vi "Calc.vi"(1 "y":sgl, 2 "x":sgl, 3 "X_r":dbl, 4 "X_l":dbl) -> ()   [LabVIEW 2012]
panel:
  out "Found?":bool
  out "MC":dbl
  out "gamma (deg)":dbl
  out "gamma (rad)":dbl
  out "MF":dbl
  in  "Set Distance [m]":dbl
  out "Beta (angle to target) [deg]":dbl
  out "cos_2alpha":dbl
  out "F_1B_1":i32
  out "s":dbl
  out "A_1F":dbl
  out "A_1B_1":dbl
  out "F_1A_1":i32
  out "Beta (rad)":dbl
  out "CF (distance to target) [m]":dbl
  # "Input"
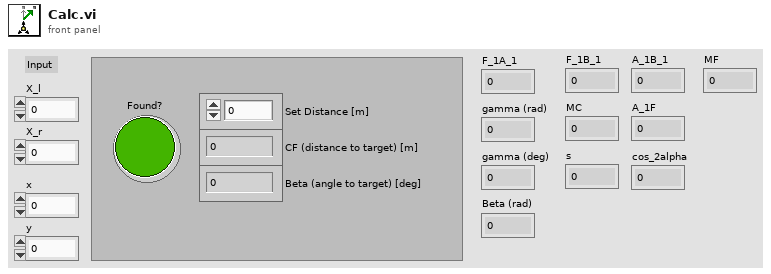
[diagram p1: front panel]
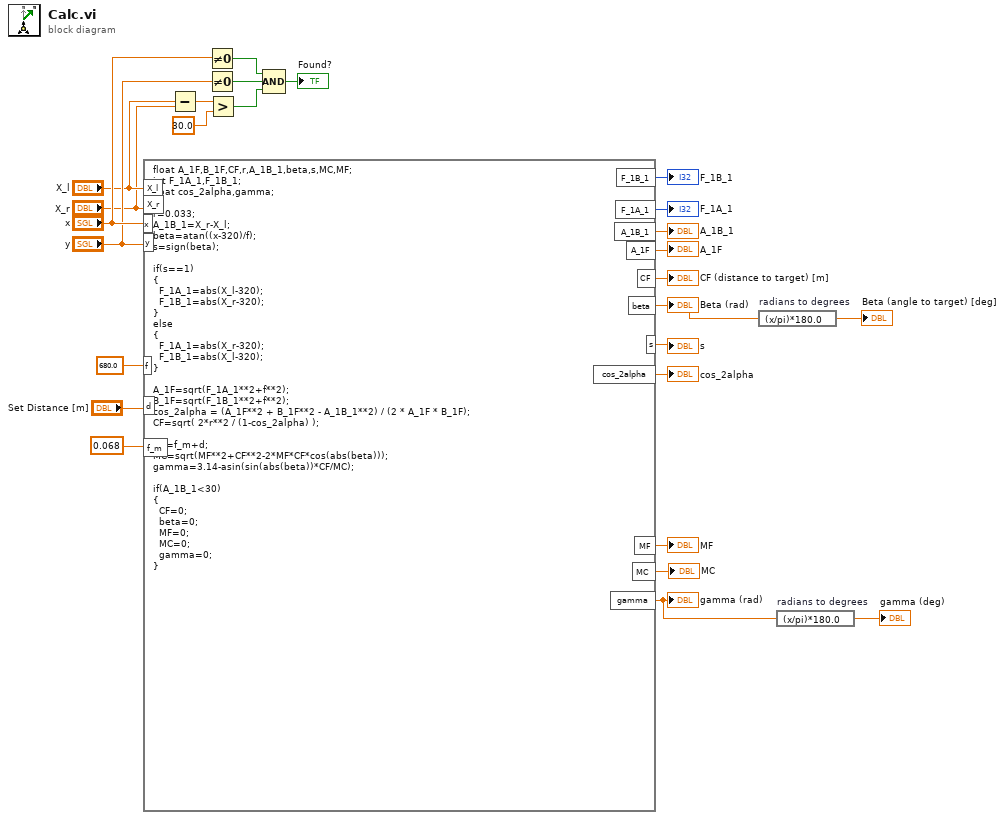
[diagram p0: block diagram]
diagram:
  n1 = formula code="float A_1F,B_1F,CF,r,A_1B_1,beta,s,MC,MF;\nint F_1A_1,F_1B_1;\nfloat cos_2alpha,gamma;\n\nr=0.033;\nA_1B_1=X_r-X_l;\nbeta=atan((x-320)/f);\ns=sign(beta);\n\nif(s==1)\n{\n  F_1A_1=abs(X_l-320);\n  F_1B_1=abs(X_r-320);\n}\nelse\n{\n  F_1A_1=abs(X_r-320);\n  F_1B_1=abs(X_l-320);\n}\n\nA_1F=sqrt(F_1A_1**2+f**2);\nB_1F=sqrt(F_1B_1**2+f**2);\ncos_2alpha = (A_1F**2 + B_1F**2 - A_1B_1**2) / (2 * A_1F * B_1F);\nCF=sqrt( 2*r**2 / (1-cos_2alpha) );\n\nMF=f_m+d;\nMC=sqrt(MF**2+CF**2-2*MF*CF*cos(abs(beta)));\ngamma=3.14-asin(sin(abs(beta))*CF/MC);\n\nif(A_1B_1<30)\n{\n  CF=0;\n  beta=0;\n  MF=0;\n  MC=0;\n  gamma=0;\n}"("X_l"="X_l", "X_r"="X_r", "x"="x", "y"="y", "f"=680.0 ("input variable"), "d"="Set Distance [m]", "f_m"=0.068 ("input variable")) -> ("CF"=→"CF (distance to target) [m]":dbl, "beta"=w20:dbl, "F_1A_1"=→"F_1A_1":i32, "A_1B_1"=→"A_1B_1":dbl, "A_1F"=→"A_1F":dbl, "s"=→"s":dbl, "F_1B_1"=→"F_1B_1":i32, "cos_2alpha"=→"cos_2alpha":dbl, "MF"=→"MF":dbl, "gamma"=w15:dbl, "MC"=→"MC":dbl)
  "Beta (rad)" <- w20
  "gamma (rad)" <- w15
  n2 = Subtract(x="X_l", y="X_r") -> (x-y=w8:dbl)
  n3 = Not Equal To 0?(x="x") -> (x != 0?=w4:bool)
  n4 = Not Equal To 0?(x="y") -> (x != 0?=w3:bool)
  n5 = Greater?(x=w8, y=30.0) -> (0:w2:bool)
  n6 = Compound Arithmetic op=AND(w4, w3, w2) -> (→"Found?":bool)
  n7 = expression code="(x/pi)*180.0" "radians to degrees"(w20) -> (→"Beta (angle to target) [deg]":dbl)
  n8 = expression code="(x/pi)*180.0" "radians to degrees"(w15) -> (→"gamma (deg)":dbl)
